vi "Set Custom Device Name.vi"(8 "error in":errorcluster, 10 "XML Node":refnum<k20>, 11 "Custom Device Config Ref in":refnum<data-value>) -> (0 "error out":errorcluster, 3 "Custom Device Config Ref out":refnum<data-value>)   [LabVIEW 2024, in "Config File Parser.lvlib" / "Custom Device Config.lvclass"]
uses:
  Custom Device Config.lvclass
  Custom Device Config.lvclass/Custom Device Config.ctl
  <vilib>/xml/NI_XML.lvlib
  <vilib>/xml/Close Reference(Node).vi
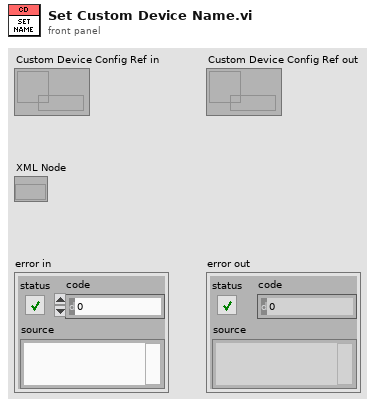
[diagram p1: front panel]
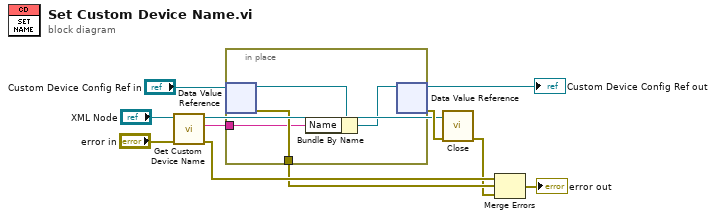
[diagram p0: block diagram]
diagram:
  n1 = call "Get Custom Device Name.vi"("error in"="error in", "XML Node"="XML Node") -> ("error out"=w10:errorcluster, "Custom Device Name"=w1:string, "XML Node out"=w2:refnum<k20>)  [unwired: 7 in]
  n2 = in-place "In Place Element Structure" {
    in-place-border: [w15] -> w9
    in-place-border: w1 -> [w12]
    n3 = in-place-dvr #1("Custom Device Config Ref in") -> (w14:refnum<class "Custom Device Config.lvclass">, w15:errorcluster)
    n4 = Bundle By Name(cluster=w14, "Name"=w12) -> (w13:refnum<class "Custom Device Config.lvclass">)
    n5 = in-place-dvr #1(w13) -> (→"Custom Device Config Ref out":refnum<data-value>, w7:errorcluster)
  }
  n6 = call-poly <vilib>:"Close.vi"("error in (no error)"=w7, "node"=w2) -> ("error out"=w6:errorcluster)  [unwired: 7 in]
  n7 = Merge Errors(w10, w9, w6) -> (→"error out":errorcluster)
